vi "2 ^ n Reduction.vi"(1 "64b (s-fxp-47) in":fxp<+/-,64,47>, 2 "N":fxp<+,6,6>) -> (0 "18b (s-fxp-1) out":fxp<+/-,18,1> format="%.18g")   [LabVIEW 2009]
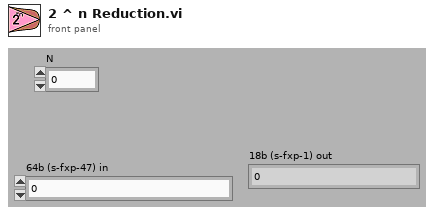
[diagram p1: front panel]
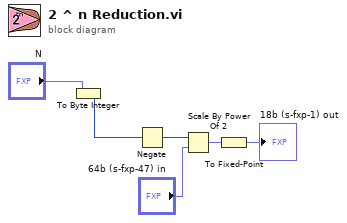
[diagram p0: block diagram]
diagram:
  n1 = To Byte Integer(number="N") -> (8bit integer=w1:i8)
  n2 = Negate(x=w1) -> (-x=w2:i8)
  n3 = Scale By Power Of 2(n=w2, x="64b (s-fxp-47) in") -> (x*2^n=w3:fxp<+/-,64,47>)
  n4 = To Fixed-Point(number=w3) -> (fixed-point=→"18b (s-fxp-1) out":fxp<+/-,18,1>)  [unwired: 1 in]
